vi "Create.vi"(5 "Error In":refnum<class "Error.lvclass">, 8 "error in (no error)":errorcluster, 11 "ErrorType":T1) -> (0 "error out":errorcluster, 3 "Error":refnum<class "Error.lvclass">)   [LabVIEW 2017, in "Transparent Assertions.lvlib" / "Error.lvclass"]
uses:
  Error.lvclass
  ErrorType.ctl
  Error.lvclass/Error.ctl
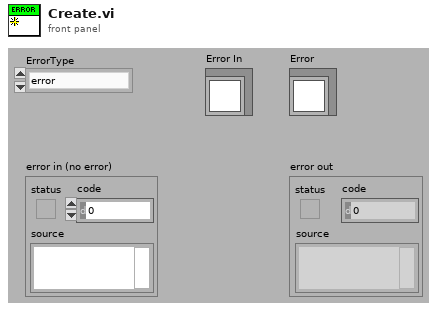
[diagram p1: front panel]
types:
  T1 = typedef "Transparent Assertions.lvlib/Error.lvclass/ErrorType.ctl" = enum16{"error", "warning", "no error"}
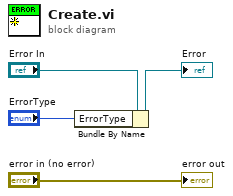
[diagram p0: block diagram]
diagram:
  n1 = Bundle By Name(cluster="Error In", "ErrorType"="ErrorType") -> (→"Error":refnum<class "Error.lvclass">)
  "error out" <- "error in (no error)"
